vi "update channel file.vi"(6 "Channel Properties File":path=path "C:/Users/User/Documents/Logs/PMT_watchlist.csv", 8 "error in":errorcluster, 9 "Value":variant, 10 "Property":T1, 11 "Channel":T2={" Card.Channel"=1.12, "Crate"=0} {"Card.Channel" format="%.2f"}) -> (0 "error out":errorcluster)   [LabVIEW 2018]
uses:
  channel.ctl
  Channel Properties.ctl
  <vilib>/Utility/file.llb/Read Delimited Spreadsheet (string).vi
  CAEN globals.vi
  dbl to fr string small.vi
  bool to string small.vi
  <vilib>/Utility/file.llb/Write Delimited Spreadsheet (string).vi
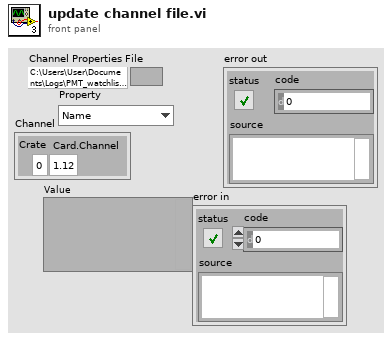
[diagram p1: front panel]
types:
  T1 = typedef "Channel Properties.ctl" = enum16{"Name", "Vset", "Vfile", "Vswmax", "Iset", "Enable", "Flag", "Vbackup"}
  T2 = typedef "channel.ctl" = cluster{" Card.Channel":dbl, "Crate":i32}
  T3 = typedef "channel_cluster.ctl" = cluster{"Channel Name":string, "Crate":i32, "Card Type":string, "Card":i32, "Channel":i32, "Status Icon":picture, "Vmon (V)":dbl, "Vset (V)":dbl, "Imon (A)":dbl, "Iset (A)":dbl, "Timestamp":string, "ON/OFF":bool, "Status":string, "Vswmax (V)":dbl, "Flag":bool, "Vfile (V)":dbl, "Error Logged":bool[], "enable_file":bool}
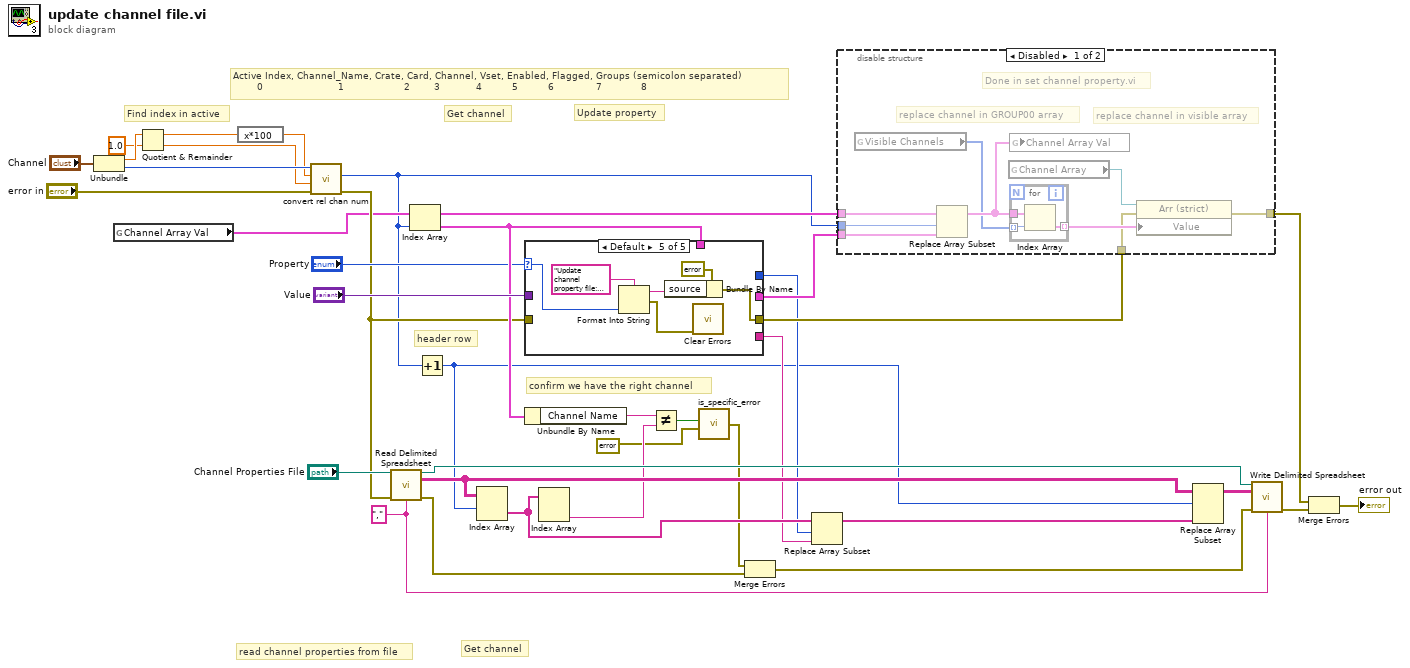
[diagram p0: block diagram]
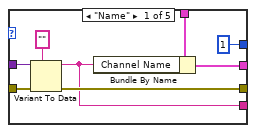
[diagram p3: hidden frame]
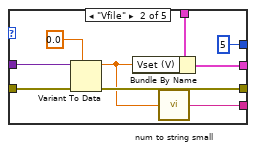
[diagram p4: hidden frame]
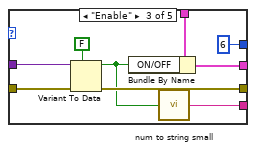
[diagram p5: hidden frame]
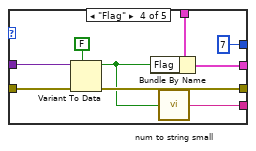
[diagram p6: hidden frame]
diagram:
  w31 = "," ("delimiter (\\t)")
  # "header row"
  # "Active Index, Channel_Name, Crate, Card, Channel, Vset, Enabled, Flagged, Groups (semicolon separated)\n        0                         1                    2        3            4          5          6              7             8"
  # "confirm we have the right channel"
  # "Get channel"
  # "read channel properties from file"
  # "Update property"
  # "Get channel"
  # "Find index in active"
  n1 = Unbundle("Channel") -> ("Card.Channel"=w11:dbl, "Crate"=w9:i32)
  n2 = global read "CAEN globals.vi" "Channel Array Val"() -> (w2:T3[])
  n3 = Quotient & Remainder(x=w11, y=1.0) -> (x-y*floor(x/y)=w5:dbl, floor(x/y)=w7:dbl)
  n4 = expression code="x*100"(w5) -> (w4:dbl)
  n5 = call "convert rel chan num.vi"("error in"="error in", "Card"=w7, "Channel"=w4, "Crate"=w9) -> ("error out"=w8:errorcluster, "Absolute index"=w1:i32)  [unwired: 4 in, 2 out]
  n6 = call-poly <vilib>:"Read Delimited Spreadsheet.vi"("file path (dialog if empty)"="Channel Properties File", "error in (no error)"=w8, "delimiter (\\t)"=w31) -> ("new file path (Not A Path if cancelled)"=w33:path, "all rows"=w34:string[][], "error out"=w18:errorcluster)  [unwired: 7 in, 3 out]
  n7 = Index Array(array=w2, index=w1) -> (element=w29:T3)
  n8 = Increment(x=w1) -> (x+1=w6:i32)
  n9 = Index Array(array=w34, index (row)=w6) -> (element=w21:string[])  [unwired: 1 in]
  n10 = case shown="Default" "Property" {
    selector: "Property" -> [_ _ _ _ w73]
    tunnel: [w44 w53 w62 w71 _] -> w36
    tunnel: "Value" -> [w43 w52 w61 w70 _]
    tunnel: w29 -> [w42 w51 w59 w68 _]
    tunnel: w8 -> [w41 w50 w58 w67 _]
    tunnel: [w40 w49 w57 w66 w76] -> w25
    tunnel: [w38 w48 w56 w65 _] -> w14
    tunnel: [1 ("index") 5 ("index") 6 ("index") 7 ("index") _] -> w13
    frame "Name" {
      n11 = Variant To Data(error in=w41, type="" ("delimiter (\\t)"), Variant=w43) -> (data=w38:string, error out=w40:errorcluster)
      n12 = Bundle By Name(cluster=w42, "Channel Name"=w38) -> (w44:T3)
    }
    frame "Vfile" {
      n13 = Variant To Data(error in=w50, type=0.0, Variant=w52) -> (data=w47:dbl, error out=w49:errorcluster)
      n14 = Bundle By Name(cluster=w51, "Vset (V)"=w47) -> (w53:T3)
      n15 = call-poly "num to string small.vi"("number"=w47) -> ("String"=w48:string)  [unwired: 14 in]
    }
    frame "Enable" {
      n16 = Variant To Data(error in=w58, type=FALSE ("Set channel property"), Variant=w61) -> (data=w55:bool, error out=w57:errorcluster)
      n17 = Bundle By Name(cluster=w59, "ON/OFF"=w55) -> (w62:T3)
      n18 = call-poly "num to string small.vi"("number"=w55) -> ("String"=w56:string)  [unwired: 14 in]
    }
    frame "Flag" {
      n19 = Variant To Data(error in=w67, type=FALSE ("Set channel property"), Variant=w70) -> (data=w64:bool, error out=w66:errorcluster)
      n20 = Bundle By Name(cluster=w68, "Flag"=w64) -> (w71:T3)
      n21 = call-poly "num to string small.vi"("number"=w64) -> ("String"=w65:string)  [unwired: 14 in]
    }
    frame Default {
      n22 = Format Into String(format string="Update channel property file: invalid property %s" ("source"), w73) -> (resulting string=w75:string, error out=w72:errorcluster)  [unwired: 2 in]
      n23 = Bundle By Name(cluster=errorcluster {"status"=TRUE, "code"=0, "source"=""} ("error in (no error)"), "source"=w75) -> (w76:errorcluster)
      n24 = call <vilib>:"Clear Errors.vi"("error in (no error)"=w72) -> ()  [unwired: 5 in, 2 out]
    }
  }
  n25 = Unbundle By Name(w29) -> ("Channel Name"=w27:string)
  n26 = Index Array(array=w21) -> (element #2=w26:string)  [unwired: 2 in, 1 out]
  n27 = Not Equal?(x=w27, y=w26) -> (x != y?=w19:bool)
  n28 = call "is_specific_error.vi"("Boolean"=w19, "error in (no error)"=errorcluster {"status"=TRUE, "code"=0, "source"="Update channel property: channel name mismatch"}) -> ("error out"=w17:errorcluster)  [unwired: 6 in]
  n29 = Merge Errors(w17, w18) -> (w16:errorcluster)
  n30 = Replace Array Subset(array=w21, new element=w14, index=w13) -> (w20:string[])
  n31 = disable-structure shown="Disabled" {
    disable-tunnel: w2 -> [w83 _]
    disable-tunnel: w36 -> [w82 _]
    disable-tunnel: w25 -> [w80 _]
    disable-tunnel: [w79 _] -> w24
    disable-tunnel: w1 -> [w78 _]
    frame Disabled {
      # "Done in set channel property.vi"
      # "replace channel in visible array"
      # "replace channel in GROUP00 array"
      n32 = global read "CAEN globals.vi" "Visible Channels"() -> (w84:i32[])
      n33 = Replace Array Subset(array=w83, new element=w82, index=w78) -> (w85:T3[])
      n34 = global read "CAEN globals.vi" "Channel Array"() -> (w81:refnum<vi>)
      n35 = global write "CAEN globals.vi" "Channel Array Val"(w85) -> ()
      n36 = for {
        tunnel: w84 -> [w88] mode=indexing
        tunnel: w85 -> [w89]
        tunnel: [w87] -> w86 mode=indexing
        n37 = Index Array(array=w89, index=w88) -> (element=w87:T3)
      }
      n38 = property class="Arr (strict)"(reference=w81, error in=w80, "Value"=w86) -> (error out=w79:errorcluster)  [unwired: 1 out]
    }
    frame Enabled {
    }
  }
  n39 = Replace Array Subset(array=w34, new element=w20, index (row)=w6) -> (w32:string[][])  [unwired: 1 in]
  n40 = call-poly <vilib>:"Write Delimited Spreadsheet.vi"("file path (dialog if empty)"=w33, "2D data"=w32, "error in (no error)"=w16, "delimiter (\\t)"=w31) -> ("error out"=w23:errorcluster)  [unwired: 10 in, 1 out]
  n41 = Merge Errors(w24, w23) -> (→"error out":errorcluster)
